vi "Controller Test Bench (3).vi"() -> ()   [LabVIEW 2022 SP3]
doc: "This example demonstrates how to continuously re-generate analog output data from a buffer in your computer's memory.\n\nRefer to your device documentation for pinouts and hardware capabilities."
uses:
  <vilib>/Utility/error.llb/DialogType.ctl
  <vilib>/DAQmx/configure/timing.llb/DAQmx Timing (Sample Clock).vi
  <vilib>/DAQmx/miscellaneous.llb/DAQmx Fill In Error Info.vi
  <vilib>/DAQmx/create/channels.llb/DAQmx Create Channel (AI-Acceleration-Accelerometer).vi
  <vilib>/DAQmx/create/channels.llb/DAQmx Create Channel (AI-Force-IEPE Sensor).vi
  <vilib>/DAQmx/create/channels.llb/DAQmx Create Channel (AI-Sound Pressure-Microphone).vi
  <vilib>/measure/maspectr.llb/FFT Spectrum (Mag-Phase) for 1 Chan.vi
  <vilib>/DAQmx/read.llb/DAQmx Read (Analog Wfm 1Chan NSamp).vi
  <vilib>/DAQmx/read.llb/DAQmx Read (Analog 1D Wfm NChan NSamp).vi
  WhiteNoise.ctl
  <vilib>/DAQmx/create/channels.llb/DAQmx Create Channel (AO-Voltage-Basic).vi
  <vilib>/DAQmx/write.llb/DAQmx Write (Analog 1D Wfm NChan NSamp).vi
  <resource>/objmgr/daqmx.rc
  <vilib>/measure/NI_MABase.lvlib
  <vilib>/measure/NI_MAPro.lvlib
  <vilib>/measure/maspectr.llb/FFT Spectrum (Mag-Phase) for N Chan.vi
panel:
  in  "Cluster":T2={"Seed"=0.0, "Standard Deviation"=0.2, "Reset"=FALSE, "Iterator"=1.0} {"Standard Deviation" format="%0.2p"}
  out "Time domain":waveform(dbl)[](graph)
  in  "Tab Control":T3(tab)
  out "Actual Sample Rate":dbl=1000.0 format="%0.2f"
  in  "Physical Channel(s)":tag="Dev1/ao0"
  in  "Min Voltage":dbl=-3.0
  in  "Max Voltage":dbl=3.5
  in  "Sample Clock Source":tag="OnboardClock"
  in  "Sample Rate":dbl=40000.0
  in  "Stop":bool
  in  "Number of Samples":i32=40000
  in  "Task Type":T4(tab)
  in  "Min Acceleration":dbl=-100.0
  in  "Max Acceleration":dbl=100.0
  in  "Sensitivity [mV/g]":dbl=95.4
  in  "Physical Channel":tag="Dev1/ai0"
  in  "Sample Clock Source":tag="OnboardClock"
  in  "Sample Rate":dbl=40000.0
  in  "Terminal Configuration":i32(ring)=-1 items=["default"=-1, "RSE"=10083, "NRSE"=10078, "Differential"=10106, "Pseudodifferential"=12529]
  in  "Samples per Loop":i32=40000
  in  "Max Sound Pressure Level (dB)":dbl=120.0
  in  "Sound Pressure Units":i32(ring)=10081 items=["Pascals"=10081, "From Custom Scale"=10065]
  in  "Microphone Sensitivity":dbl=10.0
  in  "Sensitivity 2":dbl=50.0
  in  "Min Force":dbl=-100.0
  in  "Max Force":dbl=100.0
  in  "Sensitivity Units  2":i32(ring)=15891 items=["mVolts/N"=15891, "mVolts/lb"=15892]
  in  "Force Units":i32(ring)=15875 items=["Newtons"=15875, "Pounds"=15876, "From Custom Scale"=10065]
  in  "Window":dbl
  out "Boolean":bool
  in  "Restart Aaveraging":bool
  in  "Stop 2":bool
  in  "Reset Averaging":bool
  # "Output"
  # "Channel Settings"
  # "Timing and\nBuffer Settings"
  # "Waveform Settings"
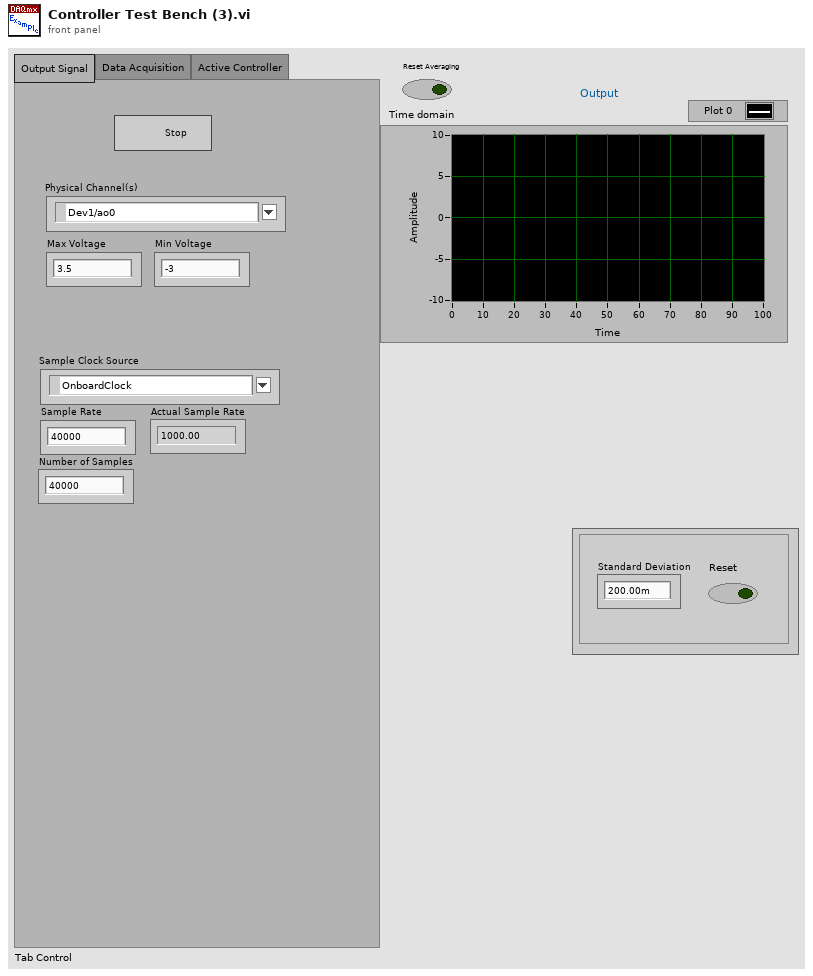
[diagram p1: front panel]
types:
  T1 = typedef "WhiteNoise.ctl" = dbl
  T2 = cluster{"Seed":T1, "Standard Deviation":dbl, "Reset":bool, "Iterator":dbl}
  T3 = enum32{"Output Signal", "Data Acquisition", "Active Controller"}
  T4 = enum32{"Acceleration", "Sound Pressure", "Force"}
  T5 = typedef "DialogType.ctl" = u16
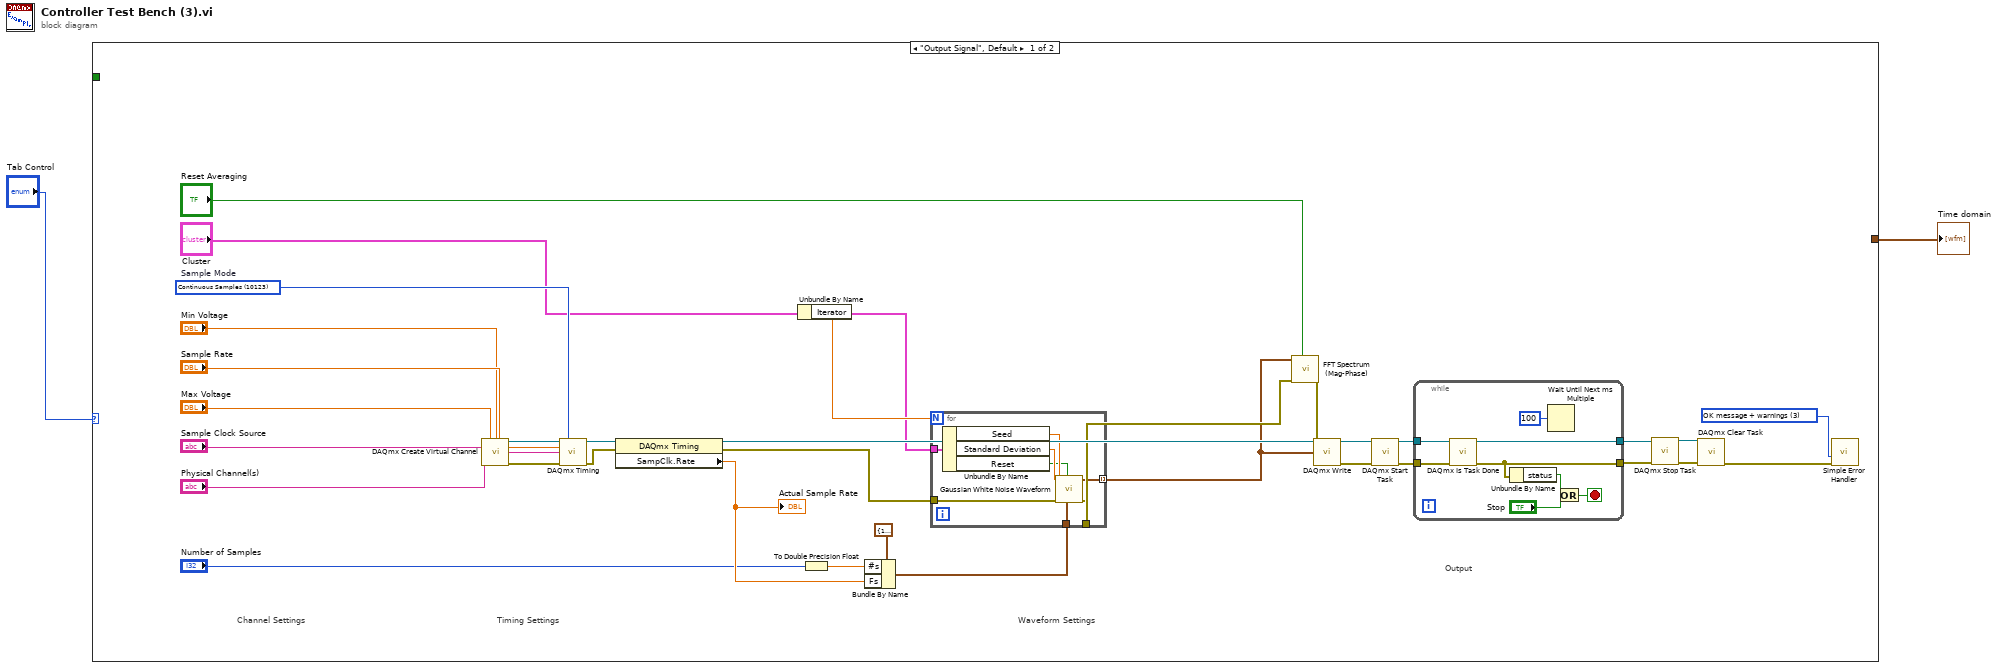
[diagram p0: block diagram]
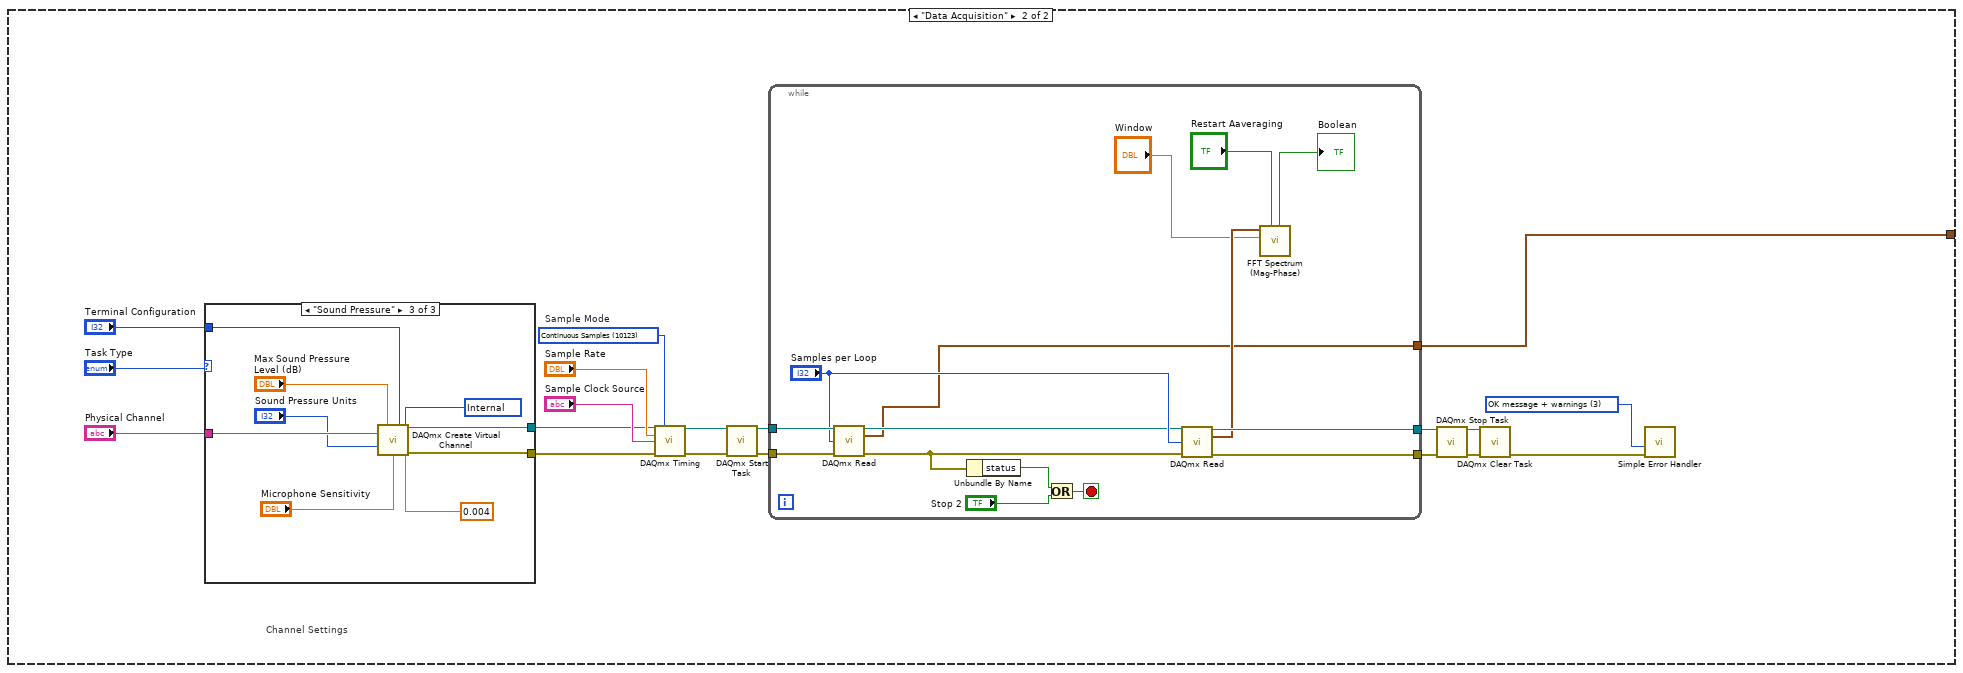
[diagram p2: hidden frame]
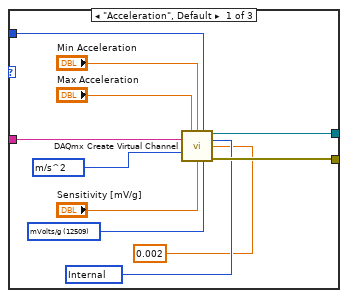
[diagram p3: hidden frame]
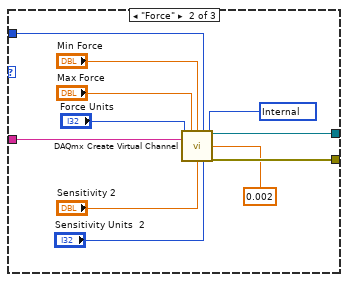
[diagram p4: hidden frame]
diagram:
  n1 = case shown="\"Output Signal\", Default" "Tab Control" {
    tunnel: [_ _] -> w2
    tunnel: [_ w53] -> w1
    frame "Output Signal", Default {
      w13 = T5 3 items=["no dialog", "OK message", "continue or stop message", "OK message + warnings", "continue/stop + warnings"] ("type of dialog (OK msg:1)")
      w34 = 10123 items=["Finite Samples"=10178, "Continuous Samples"=10123, "Hardware Timed Single Point"=12522]  # Sample Mode
      # "Output"
      # "Waveform Settings"
      # "Timing Settings"
      # "Channel Settings"
      n2 = call-poly <vilib>:"DAQmx Create Virtual Channel.vi"("maximum value"="Max Voltage", "minimum value"="Min Voltage", "physical channels"="Physical Channel(s)") -> ("task out"=w32:refnum<k21>, "error out"=w33:errorcluster)  [unwired: 11 in]
      n3 = call-poly <vilib>:"DAQmx Timing.vi"("task/channels in"=w32, "sample mode"=w34, "rate"="Sample Rate", "source"="Sample Clock Source", "error in"=w33) -> ("task out"=w36:refnum<k21>, "error out"=w35:errorcluster)  [unwired: 9 in]
      n4 = property class="DAQmx Timing"(reference=w36, error in=w35) -> (reference out=w9:refnum<k21>, error out=w8:errorcluster, "SampClk.Rate"=w22:dbl)
      "Actual Sample Rate" <- w22
      n5 = Unbundle By Name("Cluster") -> ("Iterator"=w6:dbl)
      n6 = To Double Precision Float(number="Number of Samples") -> (double precision float=w19:dbl)
      n7 = Bundle By Name(cluster=cluster{"Fs":dbl, "#s":dbl} {"Fs"=1000.0, "#s"=1000.0} ("sampling info"), "#s"=w19, "Fs"=w22) -> (w21:cluster{"Fs":dbl, "#s":dbl})
      n8 = for {
        N: w6 -> [_]
        tunnel: w8 -> [w44]
        tunnel: w21 -> [w43]
        tunnel: [w42] -> w7
        tunnel: [w41] -> w4 mode=indexing
        tunnel: "Cluster" -> [w37]
        n9 = Unbundle By Name(w37) -> ("Seed"=w40:T1, "Standard Deviation"=w39:dbl, "Reset"=w38:bool)
        n10 = call <vilib>:"Gaussian White Noise Waveform.vi"("sampling info"=w43, "reset signal"=w38, "error in (no error)"=w44, "seed"=w40, "standard deviation"=w39) -> ("error out"=w42:errorcluster, "signal out"=w41:waveform(dbl))  [unwired: 5 in]
      }
      n11 = call-poly <vilib>:"FFT Spectrum (Mag-Phase).vi"("restart averaging (F)"="Reset Averaging", "error in (no error)"=w7, "time signals"=w4) -> ("error out"=w10:errorcluster)  [unwired: 4 in, 4 out]
      n12 = call-poly <vilib>:"DAQmx Write.vi"("task/channels in"=w9, "data"=w4, "error in"=w10) -> ("task out"=w20:refnum<k21>, "error out"=w12:errorcluster)  [unwired: 10 in, 1 out]
      n13 = call <vilib>:"DAQmx Start Task.vi"("task/channels in"=w20, "error in"=w12) -> ("task out"=w31:refnum<k21>, "error out"=w30:errorcluster)  [unwired: 12 in]
      n14 = while {
        tunnel: w31 -> [w52]
        tunnel: w30 -> [w51]
        tunnel: [w48] -> w14
        tunnel: [w49] -> w15
        stop <- w50 stop-if-true
        n15 = call <vilib>:"DAQmx Is Task Done.vi"("task/channels in"=w52, "error in"=w51) -> ("task out"=w49:refnum<k21>, "error out"=w48:errorcluster)  [unwired: 11 in, 1 out]
        n16 = Unbundle By Name(w48) -> ("status"=w47:bool)
        n17 = Wait Until Next ms Multiple(millisecond multiple=u32 100) -> ()  [unwired: 1 out]
        n18 = Or(x=w47, y="Stop") -> (x .or. y?=w50:bool)
      }
      n19 = call <vilib>:"DAQmx Stop Task.vi"("task/channels in"=w15, "error in"=w14) -> ("task out"=w17:refnum<k21>, "error out"=w16:errorcluster)  [unwired: 12 in]
      n20 = call <vilib>:"DAQmx Clear Task.vi"("task in"=w17, "error in"=w16) -> ("error out"=w29:errorcluster)  [unwired: 13 in]
      n21 = call <vilib>:"Simple Error Handler.vi"("type of dialog (OK msg:1)"=w13, "error in (no error)"=w29) -> ()  [unwired: 3 in, 5 out]
    }
    frame "Data Acquisition" {
      w62 = T5 3 items=["no dialog", "OK message", "continue or stop message", "OK message + warnings", "continue/stop + warnings"] ("type of dialog (OK msg:1)")
      w71 = 10123 items=["Finite Samples"=10178, "Continuous Samples"=10123, "Hardware Timed Single Point"=12522]  # Sample Mode
      # "Channel Settings"
      n22 = case shown="\"Sound Pressure\"" "Task Type" {
        tunnel: [w91 w102 w113] -> w54
        tunnel: [w99 w110 w119] -> w65
        tunnel: "Physical Channel" -> [w98 w109 w118]
        tunnel: "Terminal Configuration" -> [w97 w108 w117]
        frame "Acceleration", Default {
          w90 = 10200 items=["Internal"=10200, "External"=10167, "None"=10230] ("IEPE Excitation Source")
          w93 = 12470 items=["g"=10186, "m/s^2"=12470, "in/s^2"=12471, "From Custom Scale"=10065] ("Acceleration Units")
          w92 = 12509 items=["mVolts/ms^2"=0, "mVolts/g"=12509, "Volts/g"=12510] ("Sensitivity Units")
          n23 = call-poly <vilib>:"DAQmx Create Virtual Channel.vi"("maximum value"="Max Acceleration", "minimum value"="Min Acceleration", "input terminal configuration"=w97, "physical channels"=w98, "current excitation source"=w90, "current excitation value"=0.002 ("IEPE Current Value (A)"), "units"=w93, "sensitivity"="Sensitivity [mV/g]", "sensitivity units"=w92) -> ("task out"=w99:refnum<k21>, "error out"=w91:errorcluster)  [unwired: 5 in]
        }
        frame "Force" {
          w100 = 10200 items=["Internal"=10200, "External"=10167, "None"=10230] ("current excitation source")
          n24 = call-poly <vilib>:"DAQmx Create Virtual Channel.vi"("maximum value"="Max Force", "minimum value"="Min Force", "input terminal configuration"=w108, "physical channels"=w109, "current excitation source"=w100, "current excitation value"=0.002, "units"="Force Units", "sensitivity"="Sensitivity 2", "sensitivity units"="Sensitivity Units  2") -> ("task out"=w110:refnum<k21>, "error out"=w102:errorcluster)  [unwired: 5 in]
        }
        frame "Sound Pressure" {
          w111 = 10200 items=["Internal"=10200, "External"=10167, "None"=10230] ("current excitation source")
          n25 = call-poly <vilib>:"DAQmx Create Virtual Channel.vi"("maximum sound pressure level"="Max Sound Pressure Level (dB)", "input terminal configuration"=w117, "physical channels"=w118, "current excitation source"=w111, "current excitation value"=0.004, "units"="Sound Pressure Units", "microphone sensitivity"="Microphone Sensitivity") -> ("task out"=w119:refnum<k21>, "error out"=w113:errorcluster)  [unwired: 7 in]
        }
      }
      n26 = call-poly <vilib>:"DAQmx Timing.vi"("task/channels in"=w65, "sample mode"=w71, "rate"="Sample Rate", "source"="Sample Clock Source", "error in"=w54) -> ("task out"=w55:refnum<k21>, "error out"=w56:errorcluster)  [unwired: 9 in]
      n27 = call <vilib>:"DAQmx Start Task.vi"("task/channels in"=w55, "error in"=w56) -> ("task out"=w60:refnum<k21>, "error out"=w59:errorcluster)  [unwired: 12 in]
      n28 = while {
        tunnel: w60 -> [w88]
        tunnel: w59 -> [w87]
        tunnel: [w83] -> w58
        tunnel: [w74] -> w57
        tunnel: [w72] -> w53
        stop <- w73 stop-if-true
        n29 = call-poly <vilib>:"DAQmx Read.vi"("task/channels in"=w88, "number of samples per channel"="Samples per Loop", "error in"=w87) -> ("task out"=w77:refnum<k21>, "data"=w72:waveform(dbl)[], "error out"=w86:errorcluster)  [unwired: 10 in]
        n30 = Unbundle By Name(w86) -> ("status"=w85:bool)
        n31 = Or(x=w85, y="Stop 2") -> (x .or. y?=w73:bool)
        n32 = call-poly <vilib>:"DAQmx Read.vi"("task/channels in"=w77, "number of samples per channel"="Samples per Loop", "error in"=w86) -> ("task out"=w83:refnum<k21>, "data"=w76:waveform(dbl), "error out"=w74:errorcluster)  [unwired: 10 in]
        n33 = call-poly <vilib>:"FFT Spectrum (Mag-Phase).vi"("restart averaging (F)"="Restart Aaveraging", "window"="Window", "time signal"=w76) -> ("phase"=w80:cluster{"f0":dbl, "df":dbl, "phase":dbl[]}, "magnitude"=w81:cluster{"f0":dbl, "df":dbl, "magnitude":dbl[]}, "averaging done"=→"Boolean":bool)  [unwired: 4 in, 2 out]
      }
      n34 = call <vilib>:"DAQmx Stop Task.vi"("task/channels in"=w58, "error in"=w57) -> ("task out"=w64:refnum<k21>, "error out"=w63:errorcluster)  [unwired: 12 in]
      n35 = call <vilib>:"DAQmx Clear Task.vi"("task in"=w64, "error in"=w63) -> ("error out"=w61:errorcluster)  [unwired: 13 in]
      n36 = call <vilib>:"Simple Error Handler.vi"("type of dialog (OK msg:1)"=w62, "error in (no error)"=w61) -> ()  [unwired: 3 in, 5 out]
    }
  }
  "Time domain" <- w1
